vi "Analog_QAM.vi"() -> ()   [LabVIEW 2014]
uses:
  <vilib>/measure/maresamp.llb/Align two Waveforms (continuous).vi
  <vilib>/express/express analysis/Spectral/Block/exnSpectralBlock spectral measurements peak poly.vi
  <vilib>/express/express analysis/Spectral/Block/exnSpectralBlock spectral measurements peak DDT.vi
  <vilib>/express/express analysis/Spectral/XNode/ExpressSpectralMeasurementsBlockNode.xnode
  <vilib>/measure/NI_MAPro.lvlib
panel:
  in  "Tab Control":enum32{"Tx", "Rx"}(tab)
  out "Transmitted Composite Signal":waveform(dbl)(graph)
  in  "I(t) Frequency":dbl=10.1 caption="Frequency"
  in  "I(t) Amplitude":dbl=1.0 caption="Amplitude"
  in  "R(t) Frequency":dbl=10.1 caption="Frequency"
  in  "R(t) Amplitude":dbl=1.0 caption="Amplitude"
  out "Modulated Signals":waveform(dbl)[](graph)
  out "Carrier":waveform(dbl)[](graph)
  in  "Carrier Amplitude":dbl=1.0 caption="Amplitude"
  in  "Carrier Frequency":dbl=10.1 caption="Frequency"
  in  "stop":bool
  out "Demodulated R(t) Signal":dynamicdata(graph)
  out "Demodulated I(t) Signal":dynamicdata(graph)
  in  "Carrier Amplitude 2":dbl=1.0 caption="Amplitude"
  in  "Carrier Frequency 2":dbl=10.1 caption="Frequency"
  in  "stop 2":bool
  out "data":dynamicdata(graph) caption="Input Signal"
  in  "Lower Cut-Off":dbl=15000.0
  in  "Upper Cut-Off":dbl=400.0
  in  "Upper Cut-Off 2":dbl=400.0 caption="Upper Cut-Off"
  in  "Lower Cut-Off 2":dbl=15000.0 caption="Lower Cut-Off"
  out "FFT of I(t)":dynamicdata(graph)
  out "FFT of R(t)":dynamicdata(graph)
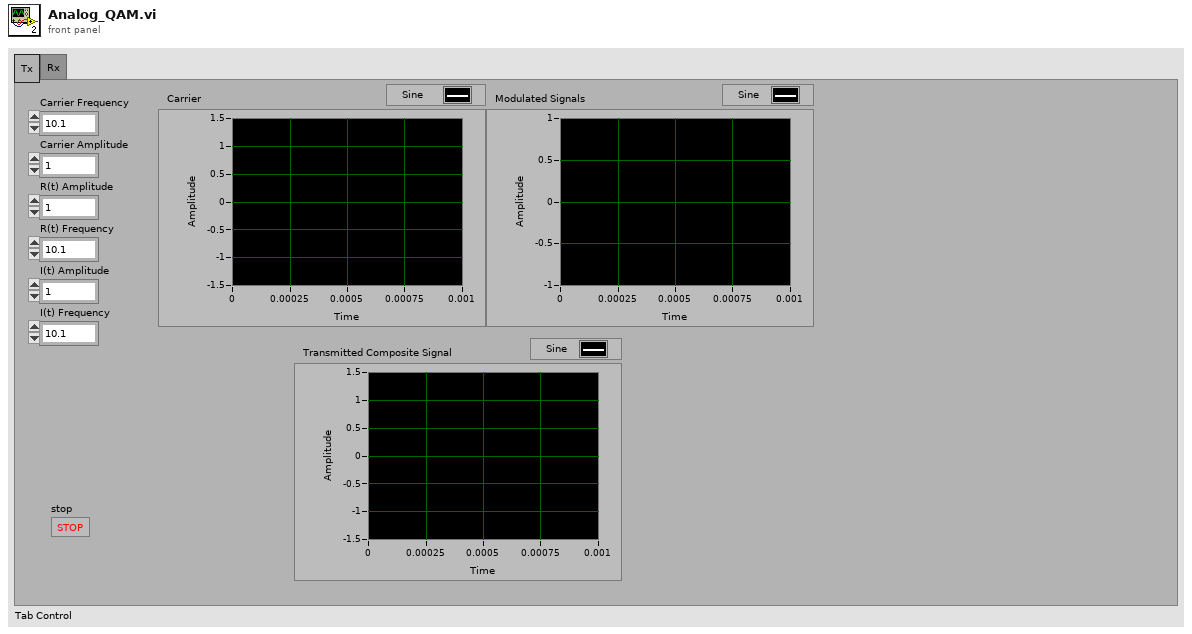
[diagram p1: front panel]
types:
  T1 = cluster{"averaging mode":u16, "weighting mode":u16, "number of averages":u32}
  T2 = cluster{"dB On (F)":bool, "unwrap phase (F)":bool, "convert to degree (F)":bool}
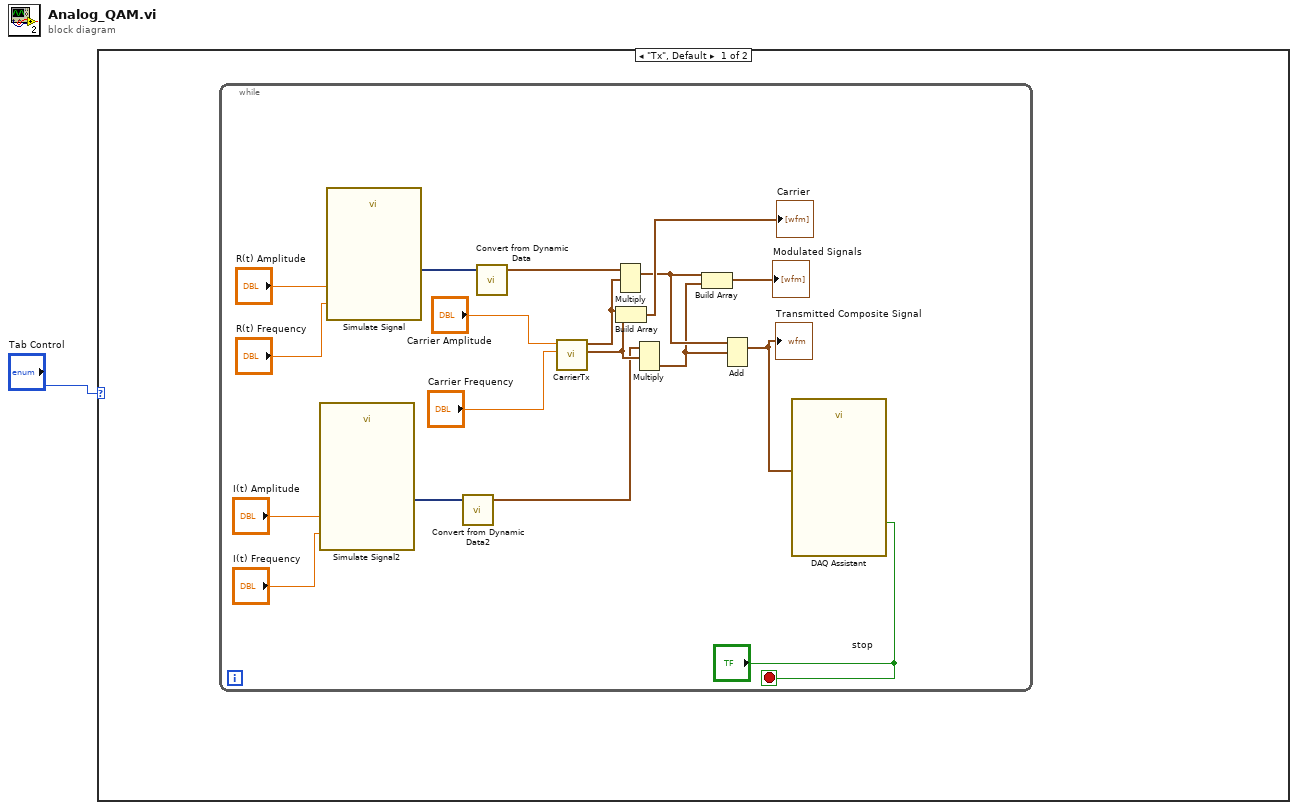
[diagram p0: block diagram]
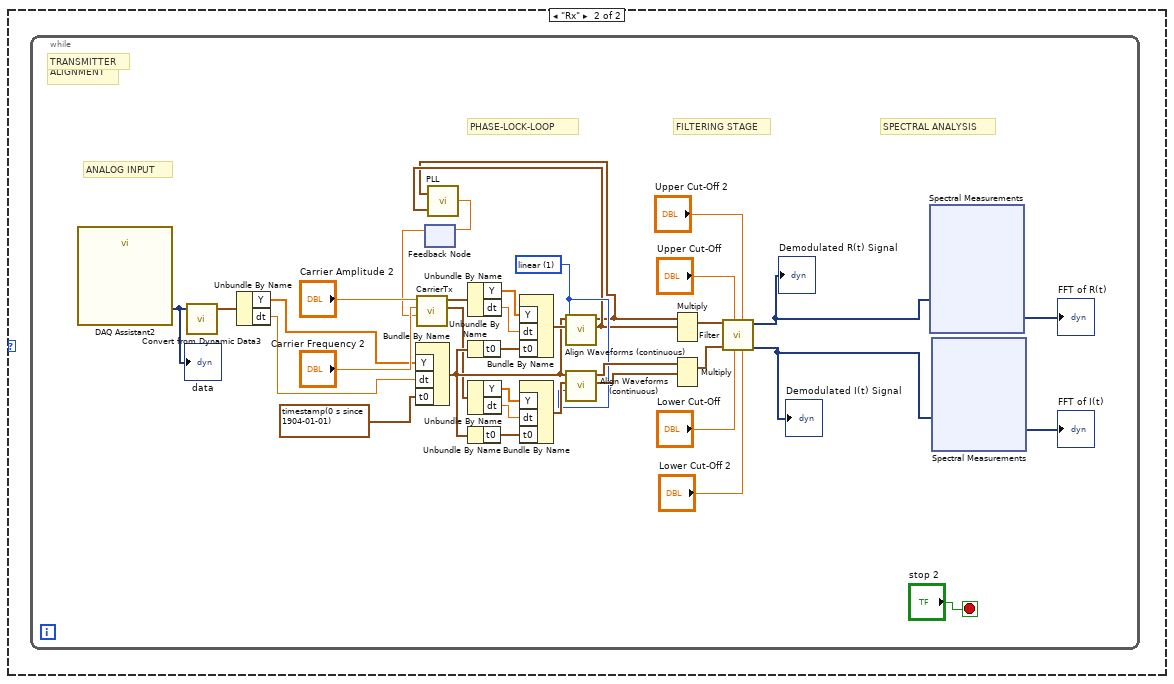
[diagram p2: hidden frame]
diagram:
  n1 = case shown="\"Tx\", Default" "Tab Control" {
    frame "Tx", Default {
      n2 = while {
        stop <- "stop" stop-if-true
        n3 = call "Simulate Signal2"("Frequency"="I(t) Frequency", "Amplitude"="I(t) Amplitude") -> ("Sine"=w11:dynamicdata)  [unwired: 12 in, 1 out]
        n4 = call "Simulate Signal"("Frequency"="R(t) Frequency", "Amplitude"="R(t) Amplitude") -> ("Sine"=w16:dynamicdata)  [unwired: 12 in, 1 out]
        n5 = call "Convert from Dynamic Data2"("Dynamic Data Type"=w11) -> ("Waveform"=w7:waveform(dbl))  [unwired: 3 in]
        n6 = call "Convert from Dynamic Data"("Dynamic Data Type"=w16) -> ("Waveform"=w15:waveform(dbl))  [unwired: 3 in]
        n7 = call "CarrierTx.vi"("Carrier Frequency"="Carrier Frequency", "Carrier Amplitude"="Carrier Amplitude") -> ("I(t) Carrier"=w8:waveform(dbl), "R(t) Carrier"=w14:waveform(dbl))  [unwired: 8 in]
        n8 = Multiply(1:w14, 2:w15) -> (0:w5:waveform(dbl))  [unwired: 1 in, 1 out]
        n9 = Build Array(w14, w8) -> (→"Carrier":waveform(dbl)[])
        n10 = Multiply(1:w8, 2:w7) -> (0:w4:waveform(dbl))  [unwired: 1 in, 1 out]
        n11 = Build Array(w5, w4) -> (→"Modulated Signals":waveform(dbl)[])
        n12 = Add(1:w4, 2:w5) -> (0:w3:waveform(dbl))  [unwired: 1 in, 1 out]
        "Transmitted Composite Signal" <- w3
        n13 = call "DAQ Assistant"("data"=w3, "stop (F)"="stop") -> ()  [unwired: 15 in, 3 out]
      }
    }
    frame "Rx" {
      n14 = while {
        stop <- "stop 2" stop-if-true
        w34 = u16 1 items=["coerce", "linear", "spline", "FIR filter"] ("interpolation mode")
        # "SPECTRAL ANALYSIS"
        # "FILTERING STAGE"
        # "PHASE-LOCK-LOOP"
        # "WAVEFORM\nALIGNMENT"
        # "ANALOG INPUT"
        # "TRANSMITTER"
        n15 = call "DAQ Assistant2"() -> ("data"=w55:dynamicdata)  [unwired: 17 in, 2 out]
        "data" <- w55
        n16 = call "Convert from Dynamic Data3"("Dynamic Data Type"=w55) -> ("Waveform"=w51:waveform(dbl))  [unwired: 3 in]
        n17 = Unbundle By Name(w51) -> ("Y"=w49:dbl[], "dt"=w48:dbl)
        n18 = Bundle By Name("Y"=w49, "dt"=w48, "t0"=timestamp(0 s since 1904-01-01)) -> (w38:waveform(dbl))  [unwired: 1 in]
        n19 = feedback #1() -> (w22:dbl)  [unwired: 1 in]
        n20 = call "CarrierTx.vi"("Phase"=w22, "Carrier Frequency"="Carrier Frequency 2", "Carrier Amplitude"="Carrier Amplitude 2") -> ("I(t) Carrier"=w37:waveform(dbl), "R(t) Carrier"=w44:waveform(dbl))  [unwired: 7 in]
        n21 = Unbundle By Name(w44) -> ("Y"=w47:dbl[], "dt"=w46:dbl)
        n22 = Unbundle By Name(w38) -> ("t0"=w45:timestamp)
        n23 = Unbundle By Name(w37) -> ("Y"=w42:dbl[], "dt"=w41:dbl)
        n24 = Unbundle By Name(w38) -> ("t0"=w40:timestamp)
        n25 = Bundle By Name("Y"=w47, "dt"=w46, "t0"=w45) -> (w43:waveform(dbl))  [unwired: 1 in]
        n26 = Bundle By Name("Y"=w42, "dt"=w41, "t0"=w40) -> (w39:waveform(dbl))  [unwired: 1 in]
        n27 = call-poly <vilib>:"Align Waveforms (continuous).vi"("interpolation mode"=w34, "waveform B in"=w43, "waveform A in"=w38) -> ("waveform B out"=w21:waveform(dbl), "waveform A out"=w20:waveform(dbl))  [unwired: 6 in, 1 out]
        n28 = call "PLL.vi"("Local Oscillator"=w21, "Input Waveform"=w20) -> ("Phase Difference"=w23:dbl)  [unwired: 1 in]
        n29 = feedback-in #1(w23) -> ()
        n30 = call-poly <vilib>:"Align Waveforms (continuous).vi"("interpolation mode"=w34, "waveform B in"=w39, "waveform A in"=w38) -> ("waveform B out"=w36:waveform(dbl), "waveform A out"=w35:waveform(dbl))  [unwired: 6 in, 1 out]
        n31 = Multiply(1:w21, 2:w20) -> (0:w31:waveform(dbl))  [unwired: 1 in, 1 out]
        n32 = Multiply(1:w36, 2:w35) -> (0:w30:waveform(dbl))  [unwired: 1 in, 1 out]
        n33 = call "Filter.vi"("Lower Cut-Off 2"="Lower Cut-Off 2", "Upper Cut-Off 2"="Upper Cut-Off 2", "Lower Cut-Off"="Lower Cut-Off", "Upper Cut-Off"="Upper Cut-Off", "Input Waveform 2"=w30, "Input Waveform"=w31) -> ("Filtered Signal 2"=w25:dynamicdata, "Filtered Signal"=w24:dynamicdata)  [unwired: 4 in]
        "Demodulated I(t) Signal" <- w25
        "Demodulated R(t) Signal" <- w24
        n34 = xnode "Spectral Measurements"("Signals"=w24) -> ("FFT - (Peak)"=→"FFT of R(t)":dynamicdata)  [unwired: 1 in, 2 out]
        n35 = xnode "Spectral Measurements"("Signals"=w25) -> ("FFT - (Peak)"=→"FFT of I(t)":dynamicdata)  [unwired: 1 in, 2 out]
      }
    }
  }
